vi "UTILITY MultiPlot.vi"(4 "Y-Axis-2":string, 6 "Y-Axis-1":string, 8 "Error In":errorcluster, 9 "X-Axis":string, 10 "Save Data":string[][](array[string]), 11 "Plot Array":dbl[][](array[numeric])) -> (0 "Error Out":errorcluster, 3 "Plot Cluster":T1(array[cluster]))   [LabVIEW 2018]
panel:
  out "subarray":string[](array[string])
  out "XY Graph":T1(graph)
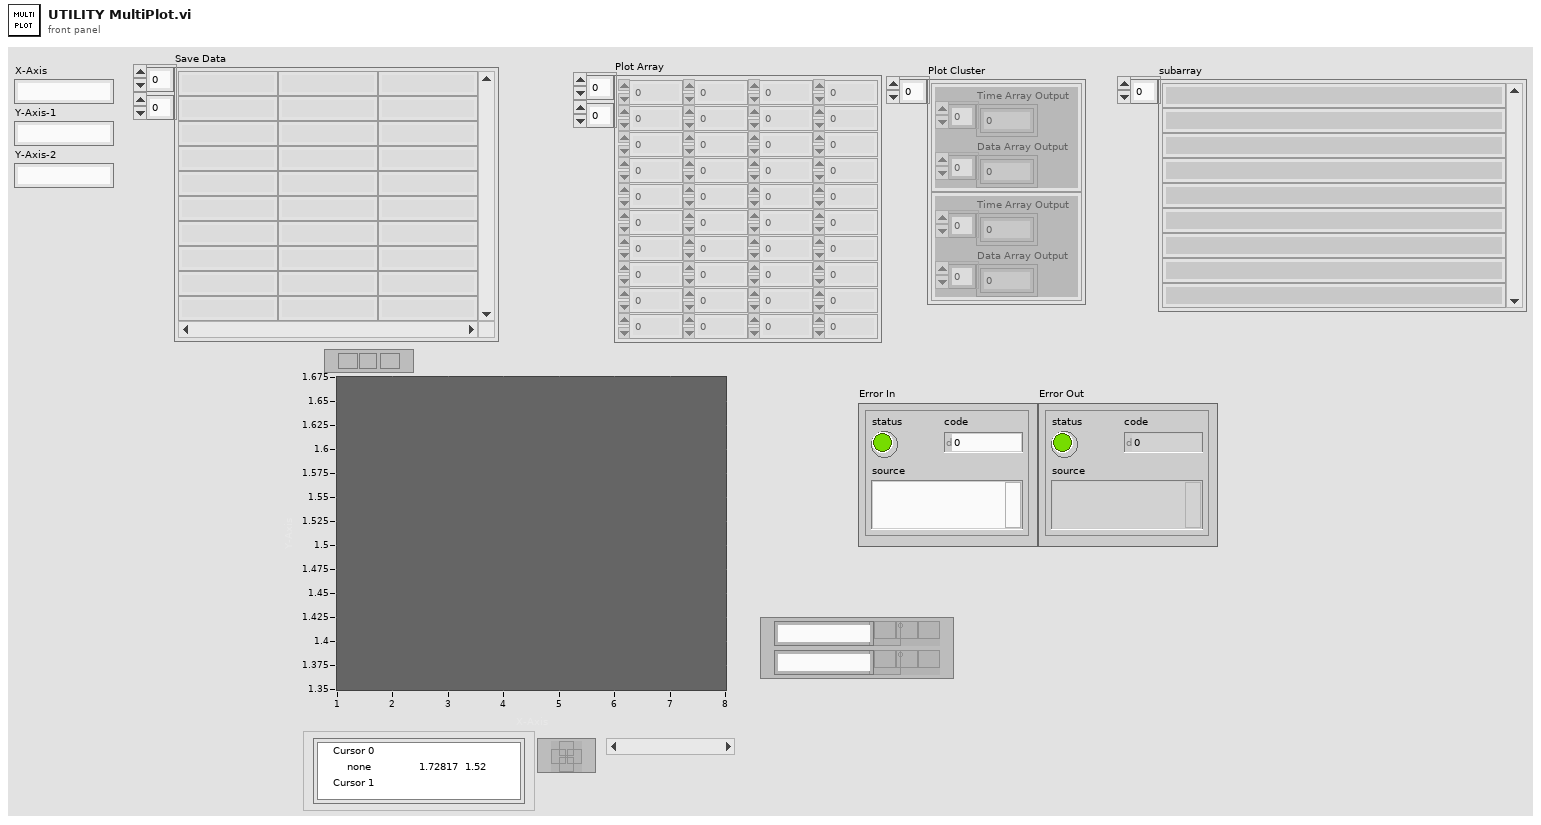
[diagram p1: front panel]
types:
  T1 = cluster{"Time Array Output":dbl[], "Data Array Output":dbl[]}[]
  T2 = cluster{"Time Array Output":dbl[], "Data Array Output":dbl[]}
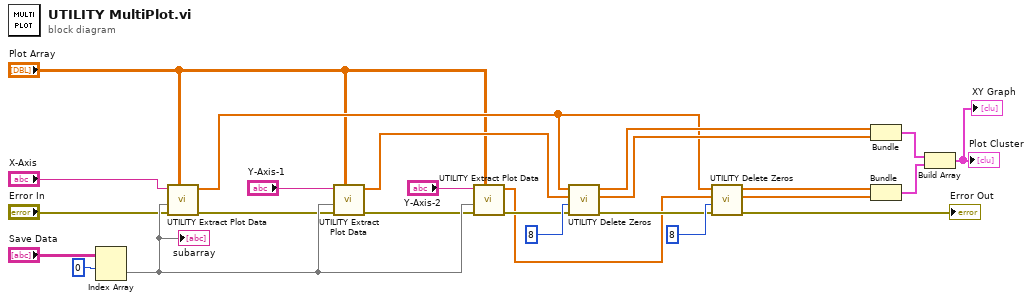
[diagram p0: block diagram]
diagram:
  n1 = Index Array(array="Save Data", index (row)=0 ("disabled index (col)")) -> (element=w9:string[])  [unwired: 1 in]
  "subarray" <- w9
  n2 = call "UTILITY Extract Plot Data.vi"("Plot Array in"="Plot Array", "Error In"="Error In", "Save Data"=w9, "Axis"="X-Axis") -> ("Error Out"=w8:errorcluster, "Plot Array out"=w18:dbl[])  [unwired: 6 in]
  n3 = call "UTILITY Extract Plot Data.vi"("Plot Array in"="Plot Array", "Error In"=w8, "Save Data"=w9, "Axis"="Y-Axis-1") -> ("Error Out"=w7:errorcluster, "Plot Array out"=w11:dbl[])  [unwired: 6 in]
  n4 = call "UTILITY Extract Plot Data.vi"("Plot Array in"="Plot Array", "Error In"=w7, "Save Data"=w9, "Axis"="Y-Axis-2") -> ("Error Out"=w5:errorcluster, "Plot Array out"=w2:dbl[])  [unwired: 6 in]
  n5 = call "UTILITY Delete Zeros.vi"("Error In"=w5, "Search # of Rows"=8, "Data Array"=w11, "Time Array"=w18) -> ("Error Out"=w4:errorcluster, "Data Array Output"=w24:dbl[], "Time Array Output"=w23:dbl[])  [unwired: 5 in]
  n6 = call "UTILITY Delete Zeros.vi"("Error In"=w4, "Search # of Rows"=8, "Data Array"=w2, "Time Array"=w18) -> ("Error Out"=→"Error Out":errorcluster, "Data Array Output"=w16:dbl[], "Time Array Output"=w17:dbl[])  [unwired: 5 in]
  n7 = Bundle("Time Array Output"=w23, "Data Array Output"=w24) -> (w15:T2)  [unwired: 1 in]
  n8 = Bundle("Time Array Output"=w17, "Data Array Output"=w16) -> (w14:T2)  [unwired: 1 in]
  n9 = Build Array(w15, w14) -> (→"Plot Cluster" →"XY Graph":T1)
